vi "Validate Selected Client Names.vi"(8 "error in (no error)":errorcluster, 10 "project ref":refnum<vi>, 11 "multicolumnListbox in":refnum<vi>) -> (0 "error out":errorcluster, 2 "warning?":bool, 3 "multicolumnListbox out":refnum<vi>)   [LabVIEW 2021, in "MeasurementClient Editor.lvlib"]
uses:
  MeasurementClient Editor.lvlib
  <vilib>/Utility/miscctls.llb/LVRowAndColumnTypeDef.ctl
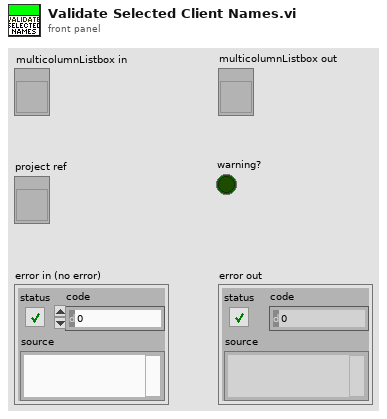
[diagram p1: front panel]
types:
  T1 = typedef "LVRowAndColumnTypeDef.ctl" = cluster{"Row":i32, "Column":i32}
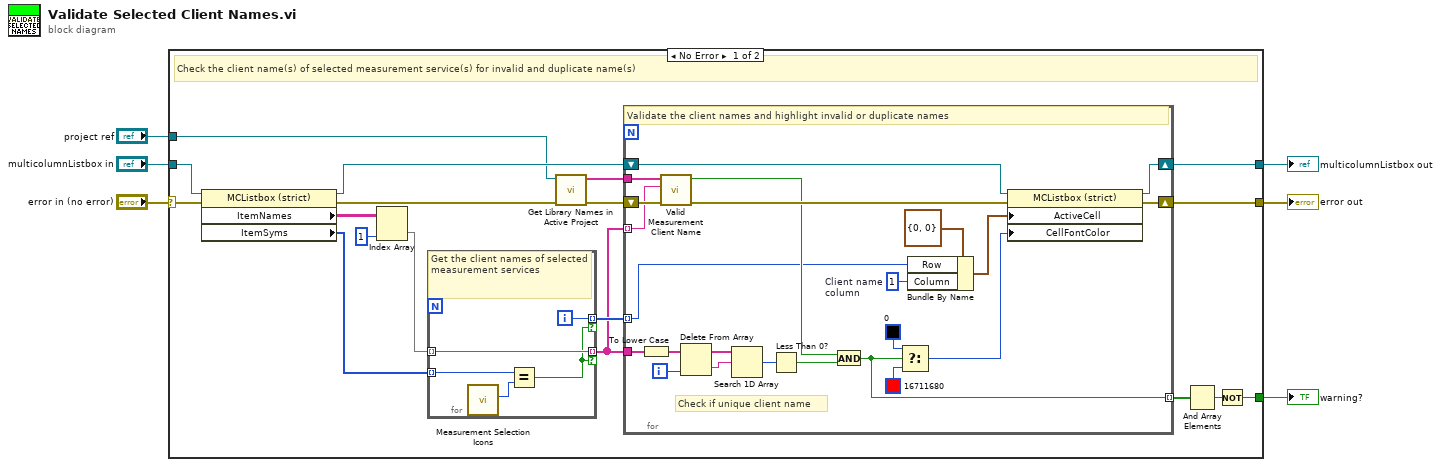
[diagram p0: block diagram]
diagram:
  n1 = case shown="No Error" "error in (no error)" {
    selector: "error in (no error)" -> [w23 w54]
    tunnel: "multicolumnListbox in" -> [w24 w53]
    tunnel: [w20 w54] -> w4
    tunnel: [w19 w53] -> w3
    tunnel: [w8 _] -> w2
    tunnel: "project ref" -> [w16 _]
    frame No Error {
      # "Check the client name(s) of selected measurement service(s) for invalid and duplicate name(s)"
      n2 = property class="MCListbox (strict)"(reference=w24, error in=w23) -> (reference out=w21:refnum<vi>, error out=w14:errorcluster, "ItemNames"=w11:string[][], "ItemSyms"=w18:i32[])
      n3 = Index Array(array=w11, index (col)=1 ("disabled index (col)")) -> (element=w13:string[])  [unwired: 1 in]
      n4 = for {
        tunnel: w13 -> [w50] mode=indexing
        tunnel: w18 -> [w52] mode=indexing
        tunnel: [w50] -> w7 mode=indexing if=w48
        tunnel: [w49] -> w12 mode=indexing if=w48
        i -> [w49]
        # "Get the client names of selected measurement services"
        n5 = call "Measurement Selection Icons.vi"() -> ("Checked"=w51:i32)  [unwired: 10 in, 1 out]
        n6 = Equal?(x=w52, y=w51) -> (x = y?=w48:bool)
      }
      n7 = call "Get Library Names in Active Project.vi"("error in (no error)"=w14, "project ref"=w16) -> ("error out"=w17:errorcluster, "library names"=w15:string[])  [unwired: 8 in]
      n8 = for {
        shift-right: [w38] -> w20
        shift-left: w17 -> [w47]
        shift-right: [w37] -> w19
        shift-left: w21 -> [w45]
        tunnel: [w31] -> w10 mode=indexing
        tunnel: w7 -> [w26]
        tunnel: w15 -> [w29]
        tunnel: w7 -> [w28] mode=indexing
        tunnel: w12 -> [w27] mode=indexing
        i -> [w25]
        w42 = 1  # Client name column
        # "Check if unique client name"
        # "Validate the client names and highlight invalid or duplicate names"
        n9 = To Lower Case(string=w26) -> (all lower case string=w30:string[])
        n10 = call "Valid Measurement Client Name.vi"("error in"=w47, "requested client name"=w28, "library names"=w29) -> ("error out"=w46:errorcluster, "valid name?"=w32:bool)  [unwired: 7 in]
        n11 = Delete From Array(array=w30, index=w25) -> (deleted portion=w35:string, array with subset deleted=w36:string[])  [unwired: 1 in]
        n12 = Search 1D Array(1D array=w36, element=w35) -> (index of element=w34:i32)  [unwired: 1 in]
        n13 = Less Than 0?(x=w34) -> (x < 0?=w33:bool)
        n14 = And(x=w32, y=w33) -> (x .and. y?=w31:bool)
        n15 = Select(t=u32 0 ("Active Cell:Cell Font:Color"), s=w31, f=u32 16711680 ("Active Cell:Cell Font:Color")) -> (s? t:f=w39:u32)
        n16 = Bundle By Name(cluster=T1 {"Row"=0, "Column"=0} ("Active Cell:Active Cell"), "Row"=w27, "Column"=w42) -> (w43:T1)
        n17 = property class="MCListbox (strict)"(reference=w45, error in=w46, "ActiveCell"=w43, "CellFontColor"=w39) -> (reference out=w37:refnum<vi>, error out=w38:errorcluster)
      }
      n18 = And Array Elements(Boolean array=w10) -> (logical AND=w9:bool)
      n19 = Not(x=w9) -> (.not. x?=w8:bool)
    }
    frame Error {
      # "Pass"
    }
  }
  "error out" <- w4
  "multicolumnListbox out" <- w3
  "warning?" <- w2
